vi "Phasor Convert phi to (m, tau).vi"(10 "Phasor Frequency":dbl[unit], 11 "Phase":dbl) -> (2 "Modulus":dbl, 3 "Phase Lifetime":dbl[unit])   [LabVIEW 2021, in "Phasor.lvlib"]
uses:
  Phasor.lvlib
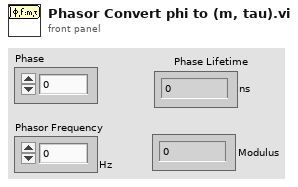
[diagram p1: front panel]
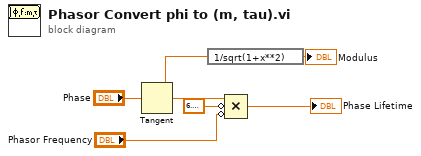
[diagram p0: block diagram]
diagram:
  n1 = Tangent(1:"Phase") -> (0:w1:dbl)
  n2 = expression code="1/sqrt(1+x**2)"(w1) -> (→"Modulus":dbl)
  n3 = Compound Arithmetic op=MULTIPLY(w1, invert 6.283185307179586, invert "Phasor Frequency") -> (→"Phase Lifetime":dbl[unit])
